vi "ROSUnregister.vi"(2 "Err in":string, 4 "Server ROS":T3={"topic port"=0, "Node"="", "topic"="", "type"="", "node port"=0, "error "={"status"=FALSE, "code"=0, "source"=""}, "Direction"=enum."Node", "APIs"=[], "Update (ms)"=1, "write queue"=1}) -> (0 "Err out":string, 1 "Log":T2)   [LabVIEW 2012]
uses:
  ROSLog.ctl
  MyState.ctl
  SubVIs/_ROSDirection.ctl
  SubVIs/_ROSControl.ctl
panel:
  out "unReply":T1
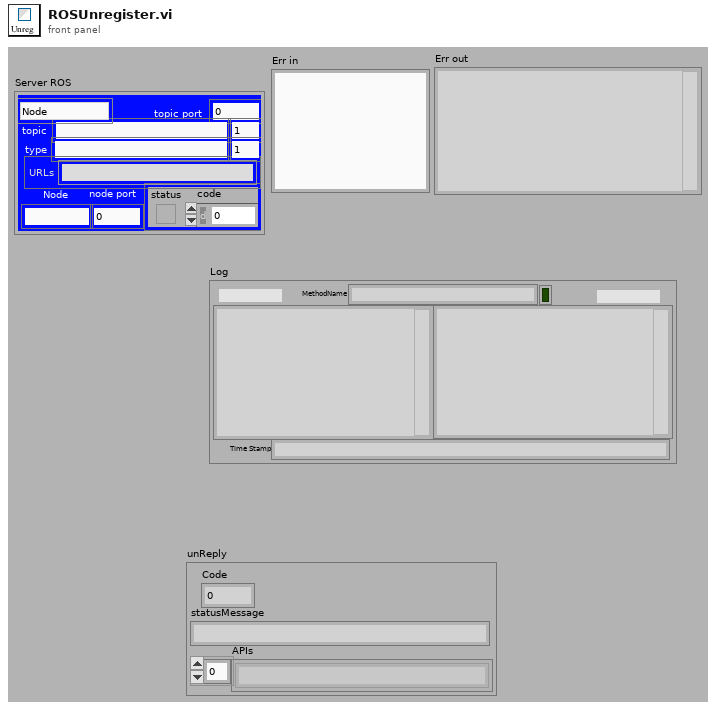
[diagram p1: front panel]
types:
  T1 = cluster{"Code":i8, "statusMessage":string, "APIs":string[]}
  T2 = typedef "ROSLog.ctl" = cluster{"Sent":string, "Reply":string, "MethodName":string, "success":bool, "Dir1":string, "Dir2":string, "Time Stamp":string}
  T3 = typedef "_ROSControl.ctl" = cluster{"topic port":u16, "Node":string, "topic":string, "type":string, "node port":u32, "error ":errorcluster, "Direction":T4, "APIs":string[], "Update (ms)":u16, "write queue":u16}
  T4 = typedef "_ROSDirection.ctl" = enum16{"Node", "Publisher", "Subscriber", "Service Client"}
  T5 = typedef "MyState.ctl" = enum16{"No Connection", "Registered", "Connected", "Close"}
  T6 = cluster{"Caller ID":string, "Topic":string, "Caller API":string}
  T7 = enum16{"http://IP:port", "http://IP", "IP:port", "IP only"}
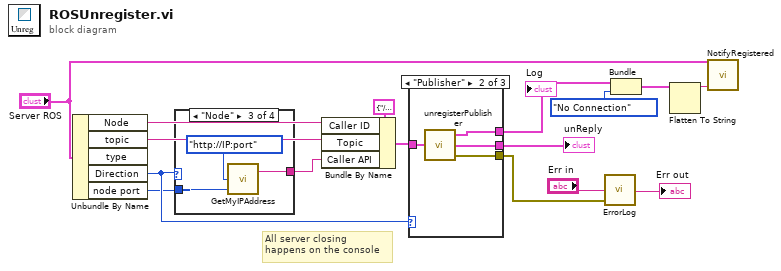
[diagram p0: block diagram]
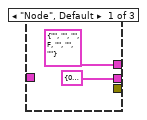
[diagram p2: hidden frame]
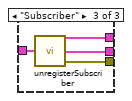
[diagram p3: hidden frame]
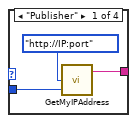
[diagram p4: hidden frame]
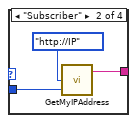
[diagram p5: hidden frame]
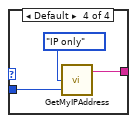
[diagram p6: hidden frame]
diagram:
  # "All server closing\nhappens on the console"
  n1 = Unbundle By Name("Server ROS") -> ("Node"=w10:string, "topic"=w11:string, "Direction"=w12:T4, "node port"=w9:u32)  [unwired: 1 out]
  n2 = case shown="\"Node\"" w12 {
    tunnel: [w19 w22 w25 w28] -> w13
    tunnel: w9 -> [w17 w20 w24 w27]
    frame "Publisher" {
      n3 = call "GetMyIPAddress.vi"("Port"=w17, "Format"=T7."http://IP:port") -> ("URI"=w19:string)  [unwired: 2 in]
    }
    frame "Subscriber" {
      n4 = call "GetMyIPAddress.vi"("Port"=w20, "Format"=T7."http://IP") -> ("URI"=w22:string)  [unwired: 2 in]
    }
    frame "Node" {
      n5 = call "GetMyIPAddress.vi"("Port"=w24, "Format"=T7."http://IP:port") -> ("URI"=w25:string)  [unwired: 2 in]
    }
    frame Default {
      n6 = call "GetMyIPAddress.vi"("Port"=w27, "Format"=T7."IP only") -> ("URI"=w28:string)  [unwired: 2 in]
    }
  }
  n7 = Bundle By Name(cluster=T6 {"Caller ID"="/labview", "Topic"="/topic", "Caller API"="API"} ("Parameters"), "Caller ID"=w10, "Topic"=w11, "Caller API"=w13) -> (w14:T6)
  n8 = case shown="\"Publisher\"" w12 {
    tunnel: w14 -> [_ w34 w38]
    tunnel: [T2 {"Sent"="", "Reply"="", "MethodName"="", "success"=FALSE, "Dir1"="", "Dir2"="", "Time Stamp"=""} ("Log") w33 w37] -> w2
    tunnel: [T1 {"Code"=0, "statusMessage"="", "APIs"=[]} ("Reply") w32 w36] -> w8
    tunnel: [_ w31 w35] -> w7
    frame "Node", Default {
    }
    frame "Publisher" {
      n9 = call "unregisterPublisher.vi"("Parameters"=w34) -> ("Error out"=w31:errorcluster, "Reply"=w32:T1, "Log"=w33:T2)  [unwired: 1 in]
    }
    frame "Subscriber" {
      n10 = call "unregisterSubscriber.vi"("Parameters"=w38) -> ("Error out"=w35:errorcluster, "Reply"=w36:T1, "Log"=w37:T2)  [unwired: 1 in]
    }
  }
  "Log" <- w2
  "unReply" <- w8
  n11 = call "ErrorLog.vi"("error in"=w7, "String in"="Err in") -> ("String out"=→"Err out":string)  [unwired: 1 in, 1 out]
  n12 = Bundle("Log"=w2, "MyState"=MyState."No Connection") -> (w4:cluster{"Log":T2, "MyState":T5})  [unwired: 1 in]
  n13 = Flatten To String(anything=w4) -> (data string=w1:string)  [unwired: 3 in, 2 out]
  n14 = call "NotifyRegistered.vi"("data string"=w1, "ROS"="Server ROS") -> ()  [unwired: 2 in]
